vi "Large int-multiply by 2.vi"(8 "error in (no error)":errorcluster, 11 "Large int (decimal)":string) -> (0 "error out":errorcluster, 2 "T = the input string contains only digits (no other characters)":bool, 3 "Large int (multiplied by 2)":string)   [LabVIEW 2021, in "Numeric Utilities.lvlib"]
uses:
  Numeric Utilities.lvlib
panel:
  out "Loop iteration":i32
  out "String (no zeroes at beginning)":string
  # "Development\ncontrols/indicators useful for development and testing, but which are not outputs of the VI"
  # "Input\nInputs to the VI"
  # "Output\nOutputs of the VI"
  # "Description\n\nBlank VI with error handling case. \n\nSummarize the use of this VI in this space."
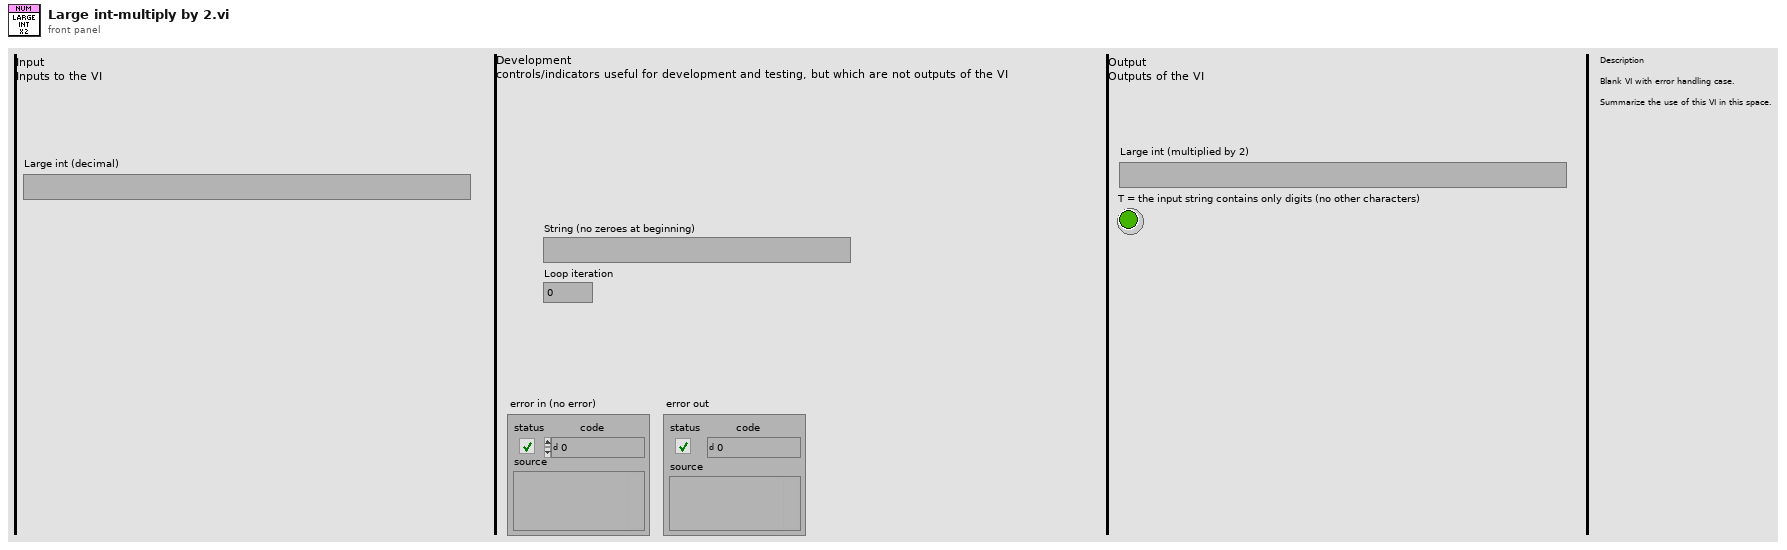
[diagram p1: front panel]
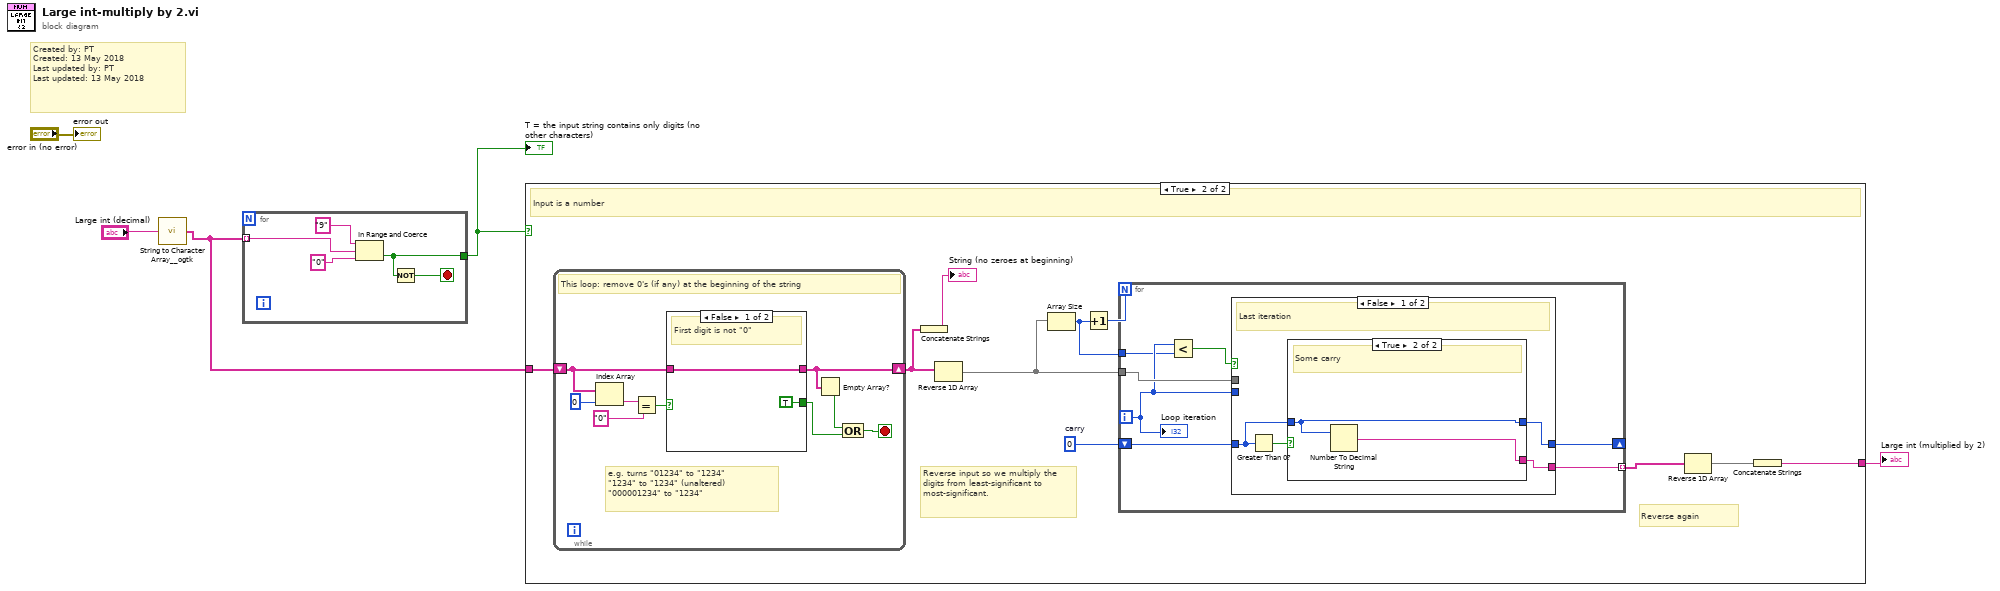
[diagram p0: block diagram]
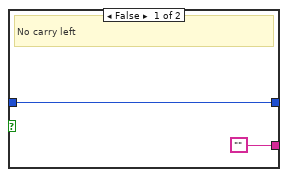
[diagram p3: hidden frame]
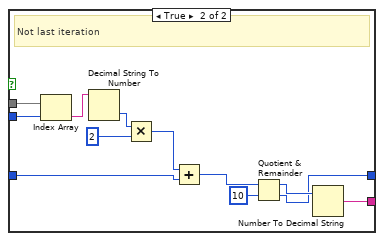
[diagram p4: hidden frame]
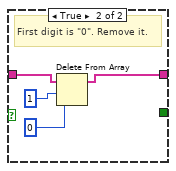
[diagram p5: hidden frame]
diagram:
  # "Created by: PT\nCreated: 13 May 2018\nLast updated by: PT\nLast updated: 13 May 2018"
  n1 = call <userlib>:"String to Character Array__ogtk.vi"("Input String"="Large int (decimal)") -> ("Character Array"=w2:string[])
  n2 = for {
    tunnel: w2 -> [w8] mode=indexing
    tunnel: [w6] -> w3
    stop <- w7 stop-if-true
    n3 = In Range and Coerce(upper limit="9", x=w8, lower limit="0") -> (In Range?=w6:bool)  [unwired: 1 out]
    n4 = Not(x=w6) -> (.not. x?=w7:bool)
  }
  "T = the input string contains only digits (no other characters)" <- w3
  n5 = case shown="True" w3 {
    tunnel: w2 -> [_ w20]
    tunnel: [_ w15] -> w1
    frame False {
      # "Input is not a number"
    }
    frame True {
      w17 = 0  # carry
      # "Reverse again"
      # "Reverse input so we multiply the digits from least-significant to most-significant."
      # "Input is a number"
      n6 = while {
        shift-right: [w50] -> w18
        shift-left: w20 -> [w53]
        stop <- w48 stop-if-true
        # "e.g. turns \"01234\" to \"1234\"\n\"1234\" to \"1234\" (unaltered)\n\"000001234\" to \"1234\""
        # "This loop: remove 0's (if any) at the beginning of the string"
        n7 = Index Array(array=w53, index=0) -> (element=w56:string)
        n8 = Equal?(x=w56, y="0") -> (x = y?=w54:bool)
        n9 = case shown="False" w54 {
          tunnel: w53 -> [w58 w62]
          tunnel: [w58 w61] -> w50
          tunnel: [TRUE _] -> w51
          frame False {
            # "First digit is not \"0\""
          }
          frame True {
            # "First digit is \"0\". Remove it."
            n10 = Delete From Array(array=w62, length=1, index=0) -> (array with subset deleted=w61:string[])  [unwired: 1 out]
          }
        }
        n11 = Empty Array?(array=w50) -> (empty?=w49:bool)
        n12 = Compound Arithmetic op=OR(w49, w51) -> (w48:bool)
      }
      n13 = Concatenate Strings(w18) -> (→"String (no zeroes at beginning)":string)
      n14 = Reverse 1D Array(array=w18) -> (reversed array=w13:string[])
      n15 = Array Size(array=w13) -> (size(s)=w11:i32)
      n16 = Increment(x=w11) -> (x+1=w12:i32)
      n17 = for {
        N: w12 -> [_]
        tunnel: w13 -> [w27]
        shift-right: [w24] -> _
        shift-left: w17 -> [w26]
        tunnel: [w25] -> w16 mode=indexing
        tunnel: w11 -> [w22]
        i -> [w23]
        n18 = Less?(x=w23, y=w22) -> (x < y?=w21:bool)
        n19 = case shown="False" w21 {
          tunnel: w27 -> [_ w47]
          tunnel: w26 -> [w28 w44]
          tunnel: [w30 w41] -> w25
          tunnel: [w29 w38] -> w24
          tunnel: w23 -> [_ w36]
          frame False {
            # "Last iteration"
            n20 = Greater Than 0?(x=w28) -> (x > 0?=w31:bool)
            n21 = case shown="True" w31 {
              tunnel: ["" w35] -> w30
              tunnel: [w32 w34] -> w29
              tunnel: w28 -> [w32 w34]
              frame False {
                # "No carry left"
              }
              frame True {
                # "Some carry"
                n22 = Number To Decimal String(number=w34) -> (decimal integer string=w35:string)  [unwired: 1 in]
              }
            }
          }
          frame True {
            # "Not last iteration"
            n23 = Index Array(array=w47, index=w36) -> (element=w37:string)
            n24 = Decimal String To Number(string=w37) -> (number=w46:i32)  [unwired: 2 in, 1 out]
            n25 = Multiply(x=w46, y=2) -> (x*y=w40:i32)
            n26 = Add(x=w40, y=w44) -> (x+y=w43:i32)
            n27 = Quotient & Remainder(x=w43, y=10) -> (x-y*floor(x/y)=w39:i32, floor(x/y)=w38:i32)
            n28 = Number To Decimal String(number=w39) -> (decimal integer string=w41:string)  [unwired: 1 in]
          }
        }
        "Loop iteration" <- w23
      }
      n29 = Reverse 1D Array(array=w16) -> (reversed array=w14:string[])
      n30 = Concatenate Strings(w14) -> (w15:string)
    }
  }
  "Large int (multiplied by 2)" <- w1
  "error out" <- "error in (no error)"
